vi "Read All Data Type Information.vi"(8 "error in (no error)":errorcluster, 11 "TwinCAT ADS in":refnum<class "TwinCAT ADS.lvclass">) -> (0 "error out":errorcluster, 1 "Data Type Information":T1[](array[typedef]) {"Category" items=["Unknown, None"=0, "Primitive"=1, "Alias"=2, "Enum"=3, "Array"=4, "Struct"=5, "FunctionBlock"=6, "Program"=7, "Function"=8, "SubRange"=9, "String"=10, "Bitset"=12, "Pointer"=13, "Union"=14, "Reference"=15, "Interface"=16]; "Type ID" items=["ADST_VOID"=0, "ADST_INT16"=2, "ADST_INT32"=3, "ADST_REAL32"=4, "ADST_REAL64"=5, "ADST_INT8"=16, "ADST_UINT8"=17, "ADST_UINT16"=18, "ADST_UINT32"=19, "ADST_INT64"=20, "ADST_UINT64"=21, "ADST_STRING"=30, "ADST_WSTRING"=31, "ADST_REAL80"=32, "ADST_BIT"=33, "ADST_MAXTYPES"=34, "ADST_BIGTYPE"=65]}, 3 "TwinCAT ADS out":refnum<class "TwinCAT ADS.lvclass">)   [LabVIEW 2018, in "TwinCAT ADS.lvclass"]
uses:
  TwinCAT ADS.lvclass
  Controls/Data Type Information.ctl
  TwinCAT.Ads
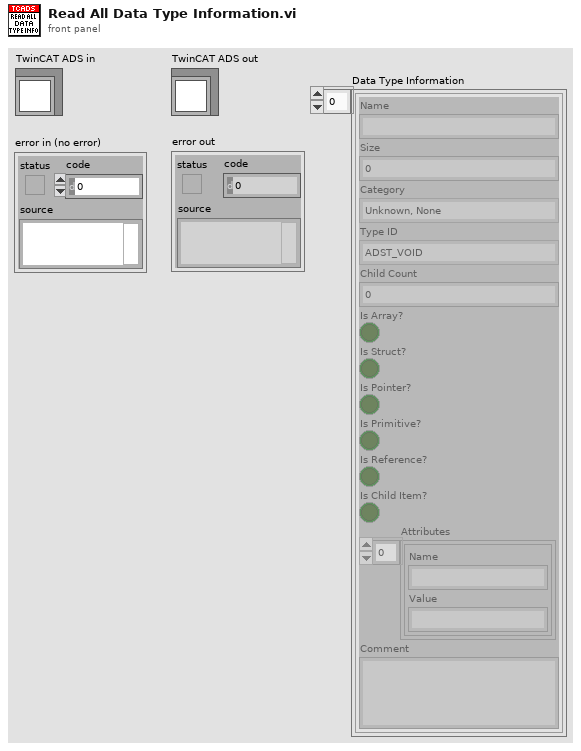
[diagram p1: front panel]
types:
  T1 = typedef "TwinCAT ADS.lvclass/Data Type Information.ctl" = cluster{"Name":string, "Size":i32, "Category":i32, "Type ID":i32, "Child Count":i32, "Is Array?":bool, "Is Struct?":bool, "Is Pointer?":bool, "Is Primitive?":bool, "Is Reference?":bool, "Is Child Item?":bool, "Attributes":cluster{"Name":string, "Value":string}[], "Comment":string}
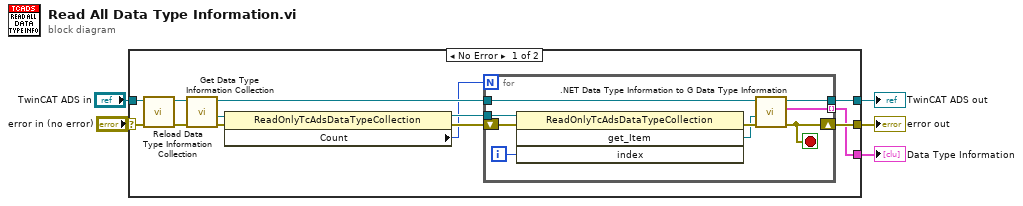
[diagram p0: block diagram]
diagram:
  n1 = case shown="No Error" "error in (no error)" {
    selector: "error in (no error)" -> [w17 w29]
    tunnel: [w13 w29] -> w4
    tunnel: [w14 w28] -> w2
    tunnel: "TwinCAT ADS in" -> [w18 w28]
    tunnel: [w12 _] -> w1
    frame No Error {
      n2 = call-dynamic "Reload Data Type Information Collection.vi"("error in (no error)"=w17, "TwinCAT ADS in"=w18) -> ("error out"=w10:errorcluster, "TwinCAT ADS out"=w11:refnum<class "TwinCAT ADS.lvclass">)  [unwired: 8 in]
      n3 = call-dynamic "Get Data Type Information Collection.vi"("error in (no error)"=w10, "TwinCAT ADS in"=w11) -> ("error out"=w8:errorcluster, "Data Type Info Collection"=w9:refnum<k24>, "TwinCAT ADS out"=w7:refnum<class "TwinCAT ADS.lvclass">)  [unwired: 7 in]
      n4 = property class="ReadOnlyTcAdsDataTypeCollection"(reference=w9, error in=w8) -> (reference out=w15:refnum<k24>, error out=w16:errorcluster, "Count"=w6:i32)
      n5 = for {
        N: w6 -> [_]
        tunnel: w15 -> [w22]
        tunnel: w7 -> [w27]
        tunnel: [w26] -> w14
        shift-right: [w25] -> w13
        shift-left: w16 -> [w23]
        tunnel: [w24] -> w12 mode=indexing
        i -> [w19]
        stop <- w25 stop-if-true
        n6 = invoke class="ReadOnlyTcAdsDataTypeCollection" method="get_Item"(reference=w22, error in=w23, "index"=w19) -> (error out=w21:errorcluster, "get_Item"=w20:refnum<k24>)  [unwired: 1 in, 2 out]
        n7 = call ".NET Data Type Information to G Data Type Information.vi"("error in (no error)"=w21, ".NET Data Type Information"=w20, "TwinCAT ADS in"=w27) -> ("error out"=w25:errorcluster, "Data Type Information"=w24:T1, "TwinCAT ADS out"=w26:refnum<class "TwinCAT ADS.lvclass">)  [unwired: 6 in]
      }
    }
    frame Error {
    }
  }
  "error out" <- w4
  "TwinCAT ADS out" <- w2
  "Data Type Information" <- w1
